vi "writePumpSpeed.vi"(8 "error in (no error)":errorcluster, 10 "Output %":dbl, 11 "Pump.Simulated in":refnum<class "Pump.Simulated.lvclass">) -> (0 "error out":errorcluster, 3 "Pump.Simulated out":refnum<class "Pump.Simulated.lvclass">)   [LabVIEW 2014, in "Pump.Simulated.lvclass"]
uses:
  Pump.Simulated.lvclass
  Pump.Simulated.lvclass/Pump.Simulated.ctl
  Pump class/Pump.lvclass
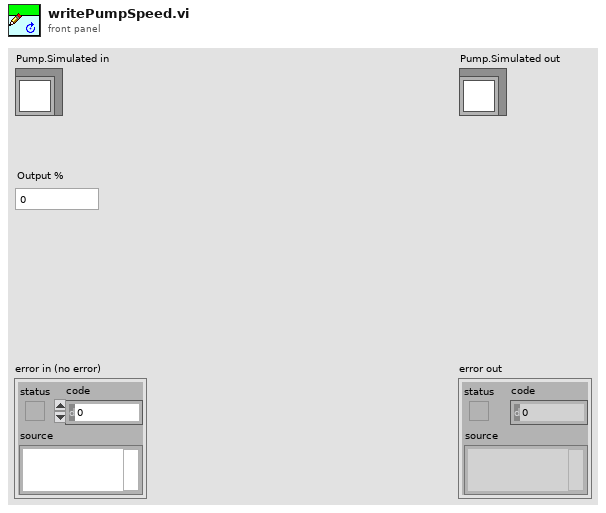
[diagram p1: front panel]
types:
  T1 = typedef "Pump.lvclass/Parameters - cluster.ctl" = cluster{"Kc":dbl, "Ti":dbl, "Td":dbl, "Min Speed":dbl, "Max Speed":dbl}
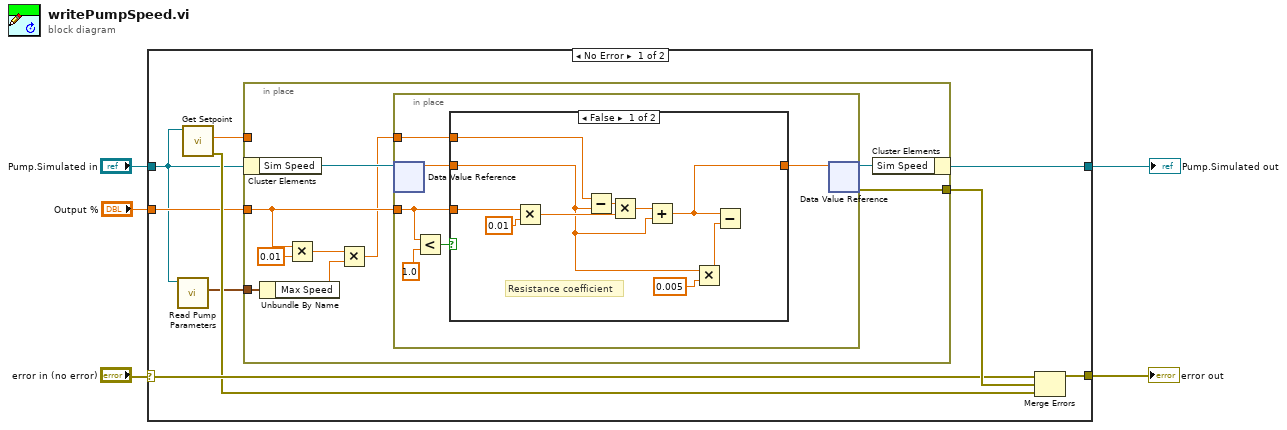
[diagram p0: block diagram]
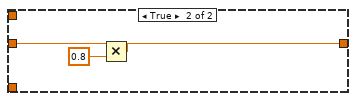
[diagram p2: hidden frame]
diagram:
  n1 = case shown="No Error" "error in (no error)" {
    selector: "error in (no error)" -> [w11 w44]
    tunnel: [w12 w44] -> w2
    tunnel: [w14 w43] -> w1
    tunnel: "Pump.Simulated in" -> [w7 w43]
    tunnel: "Output %" -> [w8 _]
    frame No Error {
      n2 = call "Read Pump Parameters.vi"("Pump in"=w7) -> ("Parameters"=w6:T1)  [unwired: 8 in, 2 out]
      n3 = call "Get Setpoint.vi"("Pump in"=w7) -> ("error out"=w10:errorcluster, "Pump Setpoint"=w9:dbl)  [unwired: 8 in, 1 out]
      n4 = in-place {
        in-place-border: [w21] -> w13
        in-place-border: w8 -> [w19]
        in-place-border: w9 -> [_]
        in-place-border: w6 -> [w17]
        n5 = in-place-cluster #1(w7) -> ("Sim Speed"=w23:refnum<data-value>)
        n6 = Unbundle By Name(w17) -> ("Max Speed"=w16:dbl)
        n7 = Multiply(x=w19, y=0.01) -> (x*y=w18:dbl)
        n8 = Multiply(x=w18, y=w16) -> (x*y=w15:dbl)
        n9 = in-place {
          in-place-border: w19 -> [w26]
          in-place-border: w15 -> [w29]
          n10 = in-place-dvr #2(w23) -> (w28:dbl)  [unwired: 1 out]
          n11 = Less?(x=w26, y=1.0) -> (x < y?=w27:bool)
          n12 = case shown="False" w27 {
            tunnel: w29 -> [w39 _]
            tunnel: [w30 w40] -> w24
            tunnel: w26 -> [w32 _]
            tunnel: w28 -> [w31 w42]
            frame False {
              # "Resistance coefficient"
              n13 = Multiply(x=w32, y=0.01) -> (x*y=w33:dbl)
              n14 = Subtract(x=w39, y=w31) -> (x-y=w37:dbl)
              n15 = Multiply(x=w37, y=w33) -> (x*y=w36:dbl)
              n16 = Add(x=w36, y=w31) -> (x+y=w30:dbl)
              n17 = Multiply(x=w31, y=0.005) -> (x*y=w34:dbl)
              n18 = Subtract(x=w30, y=w34) -> ()  [unwired: 1 out]
            }
            frame True {
              n19 = Multiply(x=w42, y=0.8) -> (x*y=w40:dbl)
            }
          }
          n20 = in-place-dvr #2(w24) -> (w22:refnum<data-value>, w21:errorcluster)
        }
        n21 = in-place-cluster #1("Sim Speed"=w22) -> (w14:refnum<class "Pump.Simulated.lvclass">)
      }
      n22 = Merge Errors(w11, w13, w10) -> (w12:errorcluster)
    }
    frame Error {
    }
  }
  "error out" <- w2
  "Pump.Simulated out" <- w1
